vi "Test External Clock2.vi"() -> ()   [LabVIEW 2021]
uses:
  Typedef/Clock Conversion.ctl
  Typedef/Timestamp Pair.ctl
  Typedef/Clock Error Statistics.ctl
  Typedef/Clock History Map.ctl
  Typedef/Clock History.ctl
  Typedef/Clock Conversion Map.ctl
  <vilib>/Platform/TimedLoop/XDataNode/timing_clust.ctl
  <vilib>/Platform/TimedLoop/XDataNode/nitl_modes.ctl
  <vilib>/Platform/TimedLoop/XDataNode/wakeup.ctl
  System Time/LabVIEW Time to TAI Time.vi
  <vilib>/numeric/sub_Random U32.vi
  SubVIs/Add Error.vi
  Errors/Append Error Location.vi
  <vilib>/Analysis/baseanly.llb/Std Deviation and Variance.vi
  <vilib>/platform/TimedLoop/XDataNode/XDataNode.xnode
  <vilib>/Platform/TimedLoop/XDataNode/XDNodeRunTimeDep.lvlib
  Time_CIF_U.lvlib
panel:
  in  "slope":dbl=1.2
  out "Error Statistics (ns)":T1
  out "Clock Conversion Array":T2[](array[typedef])
  out "error out":errorcluster
  out "Conversion error":i64
  out "Result Error (ns)":i64
  out "Error Chart 2":i64(graph)
  in  "stop":bool
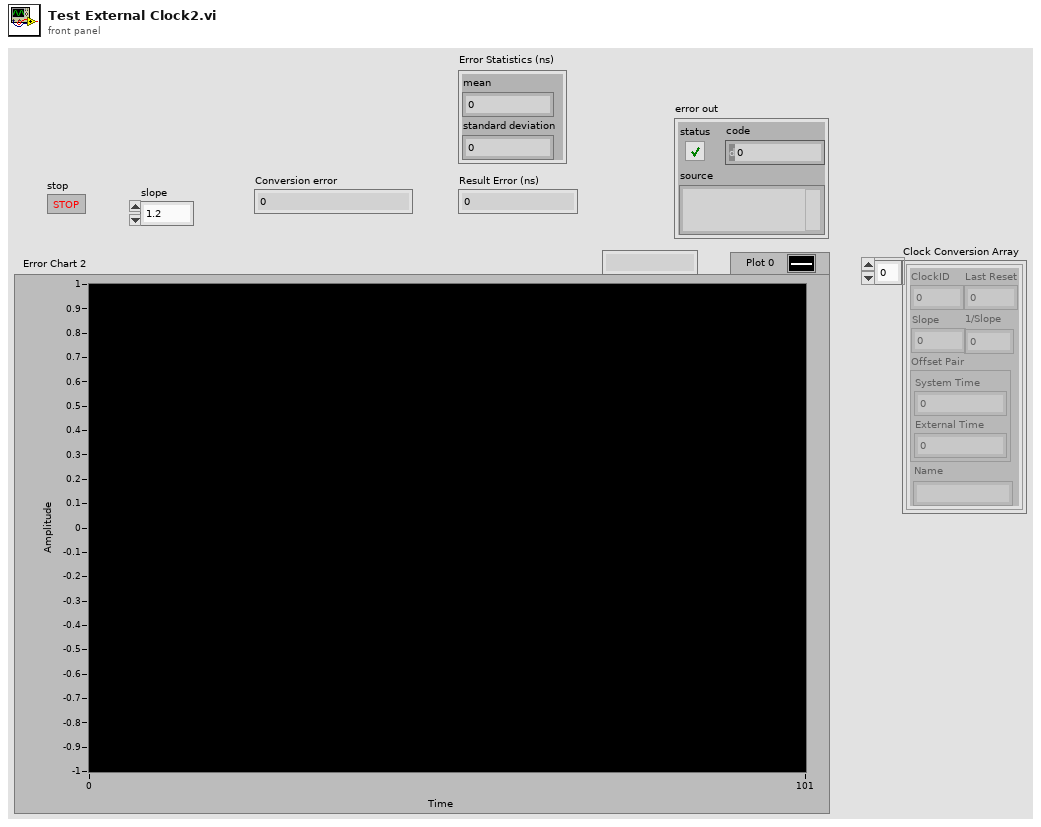
[diagram p1: front panel]
types:
  T1 = typedef "Time_CIF_U.lvlib/Clock Error Statistics.ctl" = cluster{"mean":i64, "standard deviation":i64}
  T2 = typedef "Time_CIF_U.lvlib/Clock Conversion.ctl" = cluster{"ClockID":u8, "Last Reset":i64, "Offset Pair":T3, "Slope":dbl, "1/Slope":dbl, "Name":string}
  T3 = typedef "Time_CIF_U.lvlib/Timestamp Pair.ctl" = cluster{"System Time":i64, "External Time":i64}
  T4 = typedef "Time_CIF_U.lvlib/Clock Conversion Map.ctl" = map{u8, cluster{"Last Reset":i64, "Offset Pair":T3, "Slope":dbl, "1/Slope":dbl}}
  T5 = typedef "Time_CIF_U.lvlib/Clock History Map.ctl" = map{u8, T6}
  T6 = typedef "Time_CIF_U.lvlib/Clock History.ctl" = cluster{"System Clock":i64[], "External Clock":i64[], "Last Reset Time":i64, "slope":dbl, "1/slope":dbl, "Offset Pair":T3, "Name":string}
  T7 = typedef "XDNodeRunTimeDep.lvlib/timing_clust.ctl" = cluster{"Expected End [f-1]":u64, "Actual End [f-1]":u64, "Finished Late? [f-1]":bool, "Expected End [i-1]":u64, "Actual End [i-1]":u64, "Finished Late? [i-1]":bool, "Expected Start [i]":u64, "Actual Start [i]":u64, "Expected Start [f]":u64, "Actual Start [f]":u64, "Source Name":string, "Structure Name":string, "Period":i64, "Deadline":i64, "Offset":i64, "Start":i64, "Priority":i32, "Timeout":i32, "Mode":T8, "Wakeup Reason":T9, "Error":errorcluster, "Source Type":string, "Secondary Source Type":string, "Global End Time":u64, "Global Start Time":u64, "Frame Duration":u64, "Iteration Duration":u64, "Assigned CPU":i32, "I/O Scan Engine Mode":u32}
  T8 = typedef "XDNodeRunTimeDep.lvlib/nitl_modes.ctl" = enum32{"No Change", "Process missed periods, maintain original phase", "Discard missed periods, maintain original phase", "Process missed periods, ignore original phase", "Discard missed periods, ignore original phase"}
  T9 = typedef "XDNodeRunTimeDep.lvlib/wakeup.ctl" = enum32{"Normal", "Aborted", "Asynchronous wakeup", "Timing source error", "Timed loop error", "Timeout"}
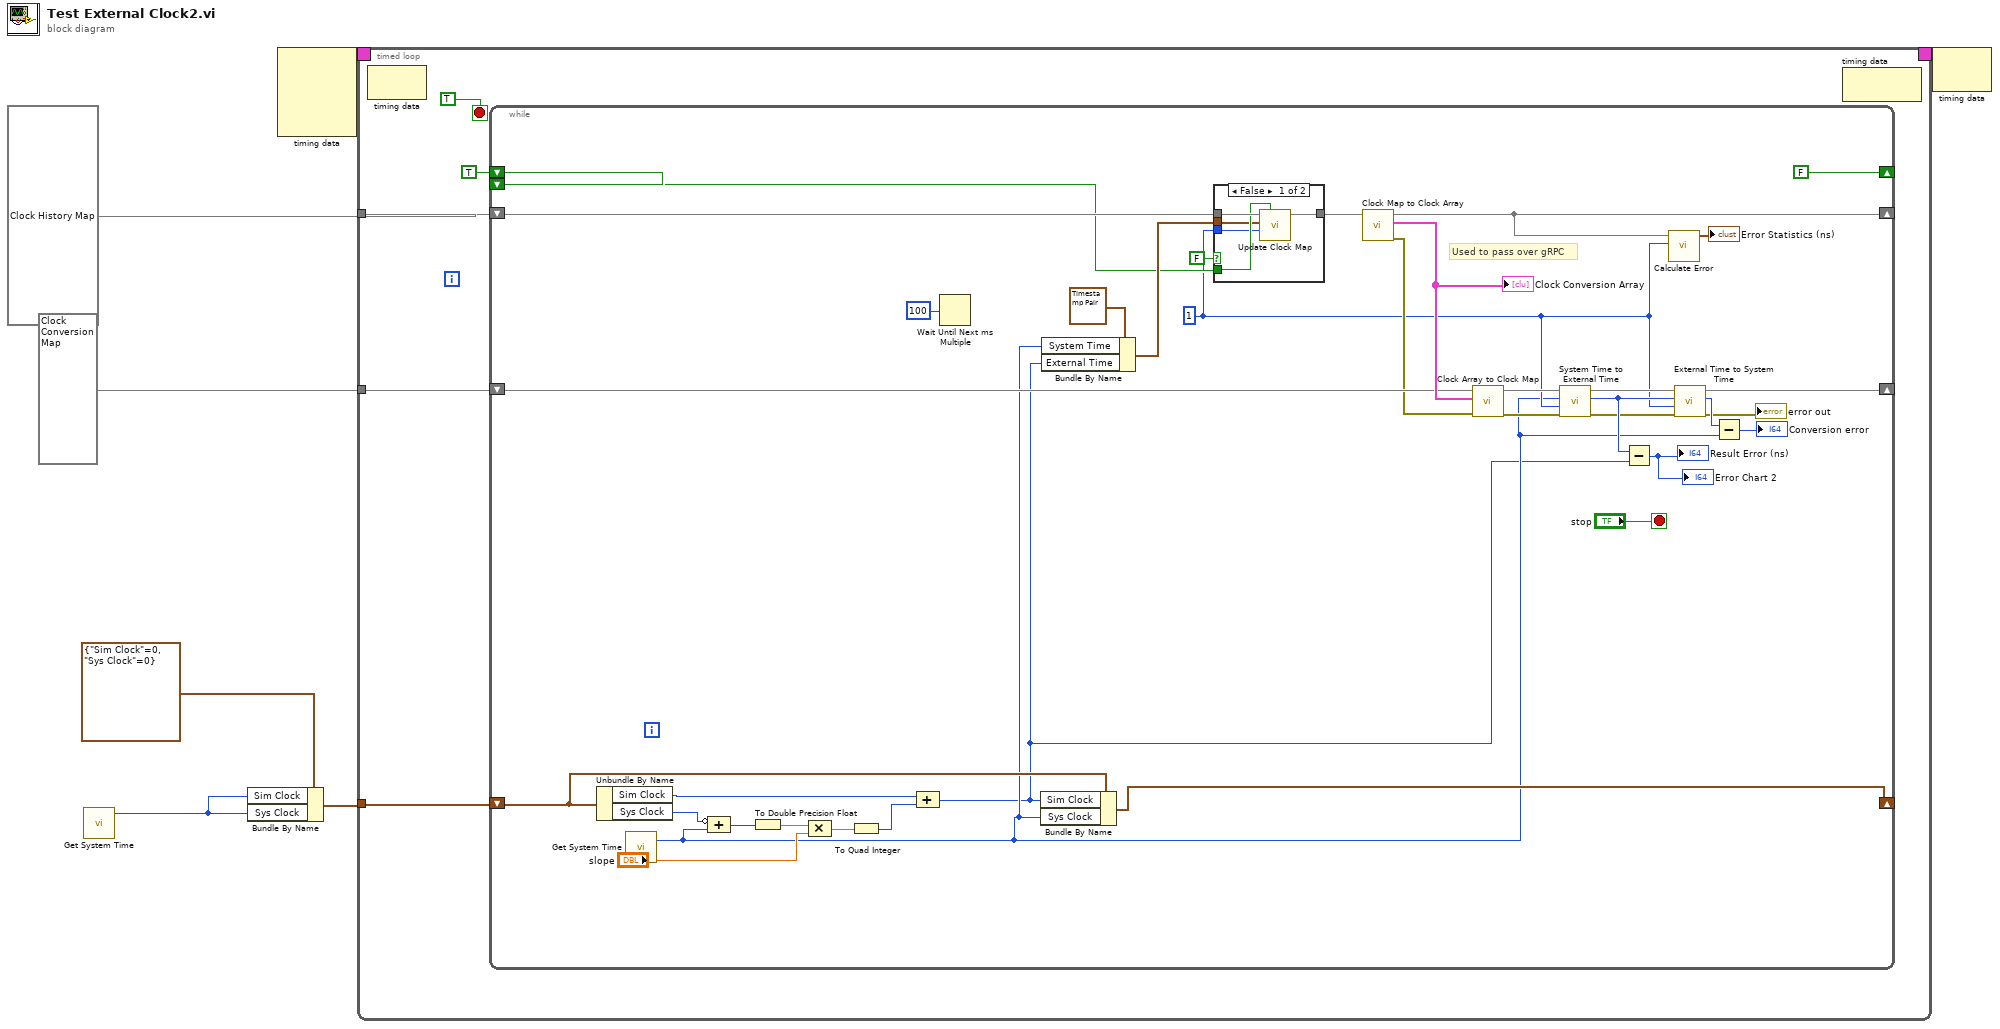
[diagram p0: block diagram]
diagram:
  n1 = call "Get System Time.vi"() -> ("Time (ns)"=w1:i64)  [unwired: 5 in]
  n2 = Bundle By Name(cluster=cluster{"Sim Clock":i64, "Sys Clock":i64} {"Sim Clock"=0, "Sys Clock"=0}, "Sim Clock"=w1, "Sys Clock"=w1) -> (w2:cluster{"Sim Clock":i64, "Sys Clock":i64})
  n3 = node-c288() -> (w7:T7)  [unwired: 4 in]
  n4 = timed-loop {
    timing: w7 -> [_]
    timing-out: [_] -> w6
    tunnel: T5 {} ("Clock History Map in") -> [w11]
    tunnel: T4 {} ("Clock Convert Map out") -> [w9]
    tunnel: w2 -> [w8]
    stop <- TRUE stop-if-true
    w10 = TRUE
    n5 = node-c288() -> ()  [unwired: 1 in, 1 out]
    n6 = while {
      shift-right: [w27] -> _
      shift-left: w11 -> [w47]
      shift-right: [FALSE] -> _
      shift-left: w10 -> [_]
      shift-left: w10 -> [w43]
      shift-right: [w34] -> _
      shift-left: w9 -> [w33]
      shift-right: [w16] -> _
      shift-left: w8 -> [w17]
      stop <- "stop" stop-if-true
      w26 = u8 1 ("ClockID")
      # "Used to pass over gRPC"
      n7 = Unbundle By Name(w17) -> ("Sim Clock"=w18:i64, "Sys Clock"=w24:i64)
      n8 = call "Get System Time.vi"() -> ("Time (ns)"=w15:i64)  [unwired: 5 in]
      n9 = Compound Arithmetic op=ADD(invert w24, w15) -> (w23:i64)
      n10 = To Double Precision Float(number=w23) -> (double precision float=w22:dbl)
      n11 = Compound Arithmetic op=MULTIPLY(w22, "slope") -> (w20:dbl)
      n12 = To Quad Integer(1:w20) -> (0:w19:i64)
      n13 = Compound Arithmetic op=ADD(w18, w19) -> (w14:i64)
      n14 = Wait Until Next ms Multiple(millisecond multiple=u32 100) -> ()  [unwired: 1 out]
      n15 = Bundle By Name(cluster=w17, "Sim Clock"=w14, "Sys Clock"=w15) -> (w16:cluster{"Sim Clock":i64, "Sys Clock":i64})
      n16 = Bundle By Name(cluster=T3 {"System Time"=1726494902617542000, "External Time"=44044000000} ("Timestamp Pair"), "System Time"=w15, "External Time"=w14) -> (w45:T3)
      n17 = case shown="False" FALSE {
        tunnel: w47 -> [w53 w54]
        tunnel: w45 -> [w50 _]
        tunnel: [w52 w54] -> w37
        tunnel: w26 -> [w49 _]
        tunnel: w43 -> [w51 _]
        frame False {
          n18 = call "Update Clock Map.vi"("Reset"=w51, "ClockID"=w49, "Timestamp Pair"=w50, "Clock History Map in"=w53) -> ("Clock History Map out"=w52:map{u8, T6})  [unwired: 6 in, 1 out]
        }
        frame True {
        }
      }
      n19 = call "Clock Map to Clock Array.vi"("Clock History Map in"=w37) -> ("error out"=w32:errorcluster, "Clock Conversion Array"=w36:T2[], "Clock History Map out"=w27:T5)  [unwired: 8 in]
      "Clock Conversion Array" <- w36
      n20 = call "Clock Array to Clock Map.vi"("error in (no error)"=w32, "Clock Conversion Array"=w36, "Clock Convert Map in"=w33) -> ("error out"=w31:errorcluster, "Clock Convert Map out"=w35:T4)  [unwired: 7 in]
      n21 = call "System Time to External Time.vi"("error in (no error)"=w31, "ClockID"=w26, "System Time"=w15, "Clock Convert Map in"=w35) -> ("error out"=w30:errorcluster, "External Time"=w41:i64, "Clock Convert Map out"=w42:T4)  [unwired: 4 in, 1 out]
      n22 = Subtract(x=w41, y=w14) -> (x-y=→"Result Error (ns)" →"Error Chart 2":i64)
      n23 = call "Calculate Error.vi"("ClockID"=w26, "Clock History Map in"=w27) -> ("Error Statistics (ns)"=→"Error Statistics (ns)":T1)  [unwired: 8 in, 1 out]
      n24 = call "External Time to System Time.vi"("error in (no error)"=w30, "ClockID"=w26, "External Time"=w41, "Clock Convert Map in"=w42) -> ("error out"=→"error out":errorcluster, "System Time"=w40:i64, "Clock Convert Map out"=w34:T4)  [unwired: 4 in, 1 out]
      n25 = Subtract(x=w40, y=w15) -> (x-y=→"Conversion error":i64)
    }
    n26 = node-c288() -> ()  [unwired: 1 in, 1 out]
  }
  n27 = node-c288(w6) -> ()  [unwired: 1 out]
